vi "Standard Bus Controller Config.vi"(8 "error in (no error)":errorcluster) -> (0 "error out":errorcluster, 3 "Configuration":T1)   [LabVIEW 2020]
doc: "Provides standard configuration information for the Bus Controller that is not defined in the XML file."
uses:
  Bus Controller/TypeDefs/Bus Controller Configuration.ctl
  Bus Controller/TypeDefs/Bus Controller Timeout.ctl
  Bus Controller/Bus Controller.lvclass
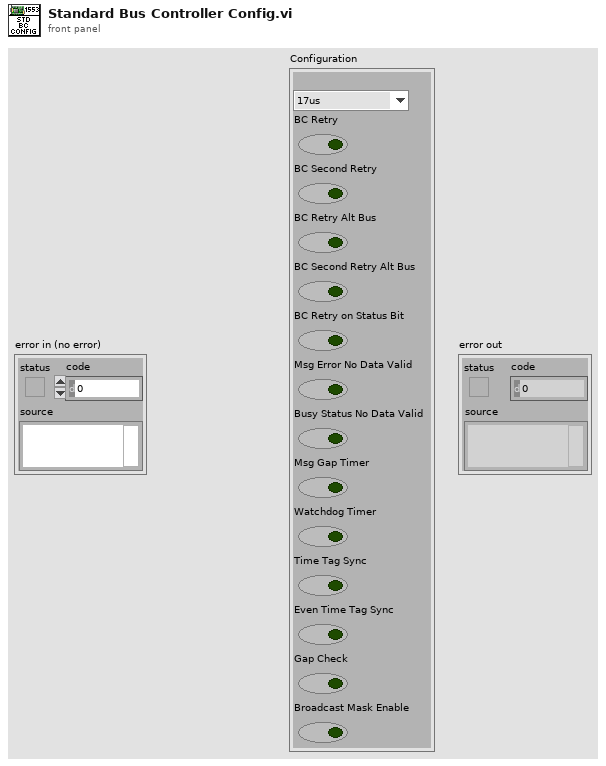
[diagram p1: front panel]
types:
  T1 = typedef "BCI-1553 API.lvlib/Bus Controller.lvclass/Bus Controller Configuration.ctl" = cluster{"Timeout":T2, "BC Retry":bool, "BC Second Retry":bool, "BC Retry Alt Bus":bool, "BC Second Retry Alt Bus":bool, "BC Retry on Status Bit":bool, "Msg Error No Data Valid":bool, "Busy Status No Data Valid":bool, "Msg Gap Timer":bool, "Watchdog Timer":bool, "Time Tag Sync":bool, "Even Time Tag Sync":bool, "Gap Check":bool, "Broadcast Mask Enable":bool}
  T2 = typedef "BCI-1553 API.lvlib/Bus Controller.lvclass/Bus Controller Timeout.ctl" = enum16{"17us", "22us", "60us", "140us"}
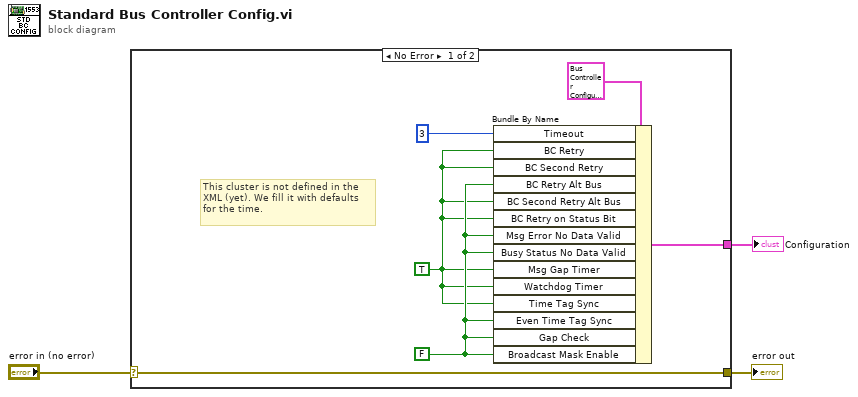
[diagram p0: block diagram]
diagram:
  n1 = case shown="No Error" "error in (no error)" {
    selector: "error in (no error)" -> [w9 w10]
    tunnel: [w9 w10] -> w2
    tunnel: [w7 _] -> w1
    frame No Error {
      w4 = TRUE ("BC Retry")
      w5 = FALSE ("BC Retry")
      # "This cluster is not defined in the\nXML (yet). We fill it with defaults\nfor the time."
      n2 = Bundle By Name(cluster=T1 {"Timeout"=enum."17us", "BC Retry"=FALSE, "BC Second Retry"=FALSE, "BC Retry Alt Bus"=FALSE, "BC Second Retry Alt Bus"=FALSE, "BC Retry on Status Bit"=FALSE, "Msg Error No Data Valid"=FALSE, "Busy Status No Data Valid"=FALSE, "Msg Gap Timer"=FALSE, "Watchdog Timer"=FALSE, "Time Tag Sync"=FALSE, "Even Time Tag Sync"=FALSE, "Gap Check"=FALSE, "Broadcast Mask Enable"=FALSE} ("Configuration"), "Timeout"=u16 3 ("BC Timeout"), "BC Retry"=w4, "BC Second Retry"=w4, "BC Retry Alt Bus"=w5, "BC Second Retry Alt Bus"=w4, "BC Retry on Status Bit"=w4, "Msg Error No Data Valid"=w5, "Busy Status No Data Valid"=w5, "Msg Gap Timer"=w4, "Watchdog Timer"=w4, "Time Tag Sync"=w4, "Even Time Tag Sync"=w5, "Gap Check"=w5, "Broadcast Mask Enable"=w5) -> (w7:T1)
    }
    frame Error {
    }
  }
  "error out" <- w2
  "Configuration" <- w1
